vi "Config.vi"(8 "error in (no error)":errorcluster, 10 "Setting":variant, 11 "Keysight 5700C in":refnum<class "Keysight 5700C.lvclass">) -> (0 "error out":errorcluster, 3 "Keysight 5700C out":refnum<class "Keysight 5700C.lvclass">)   [LabVIEW 2025, in "Power Supply.lvlib" / "Keysight 5700C.lvclass"]
uses:
  Keysight 5700C.lvclass
  Keysight 5700C.lvclass/Keysight 5700C.ctl
  PS Channel/Power Supply Channel.lvclass
  PS Channel configuration/Power Supply Channel configuration.lvclass
  Users/Public/Documents/Sandia National Labs/TSS Plugin/Abstract Engine.lvlibp/Plugin/Abstract/Abstract Instrument/Channel.ctl
  Users/Public/Documents/Sandia National Labs/TSS Plugin/Abstract Engine.lvlibp/Plugin/Abstract/Abstract Instrument/Abstract Instrument.lvclass
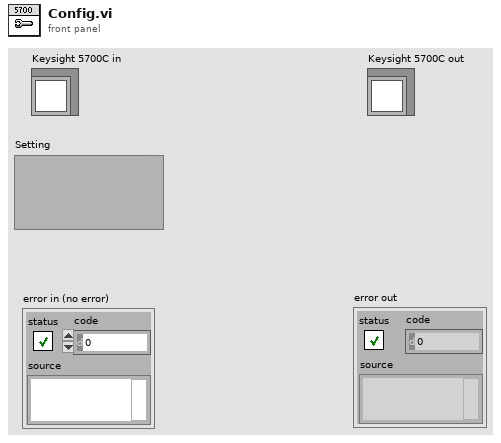
[diagram p1: front panel]
types:
  T1 = typedef "Abstract Engine.lvlibp/Abstract Instrument.lvclass/Channel.ctl" = cluster{"Alias":string, "DataType":enum16{"Anaolg Input", "Waveform"}, "Unit":enum16{"---", "V", "A", "Ohm", "Hz", "uF", "degC", "deg"}, "Upper limit":dbl, "Lower limit":dbl, "Measurement":variant}
  T2 = typedef "Abstract Engine.lvlibp/Channel configuration.lvclass/Default Channel.ctl" = cluster{"Address":string, "SW Alias":string, "Enabled":bool, "Type":string, "Description":string}
  T3 = typedef "Power Supply.lvlib/Power Supply Channel configuration.lvclass/PS Channel Setting.ctl" = cluster{"Driver":string, "Pin":string, "Test Voltage":string, "Voltage Low":dbl, "Voltage Norminal":dbl, "Voltage High":dbl, "PreTest Voltage":dbl, "PreTest Current":dbl, "Current Limit":dbl}
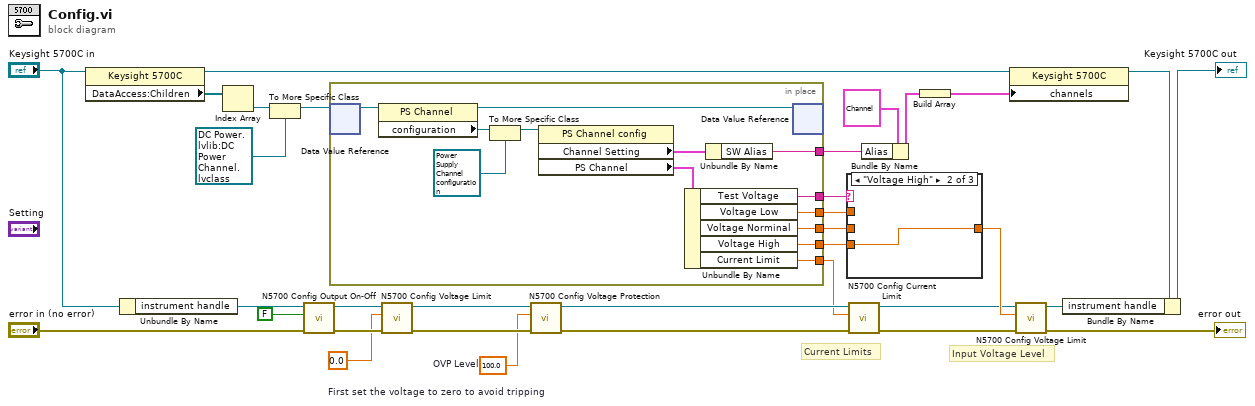
[diagram p0: block diagram]
diagram:
  w16 = 100.0  # OVP Level
  w20 = 0.0  # First set the voltage to zero to avoid tripping
  # "Input Voltage Level"
  # "Current Limits"
  n1 = property class="Keysight 5700C"(reference="Keysight 5700C in") -> (reference out=w29:refnum<class "Keysight 5700C.lvclass">, "DataAccess:Children"=w18:refnum<data-value>[])  [unwired: 1 in, 1 out]
  n2 = Unbundle By Name("Keysight 5700C in") -> ("instrument handle"=w32:refnum<visa-resource-name>)
  n3 = Index Array(array=w18) -> (element=w17:refnum<data-value>)  [unwired: 1 in]
  n4 = To More Specific Class(target class=refnum<data-value> refnum ("data value reference"), reference=w17) -> (specific class reference=w27:refnum<data-value>)  [unwired: 1 in, 1 out]
  n5 = call <instrlib>:"N5700 Config Output On-Off.vi"("error"="error in (no error)", "Output ON"=FALSE ("enabled (True)"), "VISA"=w32) -> ("error out"=w21:errorcluster, "VISA out"=w25:refnum<visa-resource-name>)  [unwired: 4 in]
  n6 = in-place {
    in-place-border: [w39] -> w13
    in-place-border: [w38] -> w12
    in-place-border: [w37] -> w11
    in-place-border: [w36] -> w10
    in-place-border: [w35] -> w9
    in-place-border: [w34] -> w8
    # "Initialize the front panel controls when loaded"
    n7 = in-place-dvr #1(w27) -> (w46:refnum<class "Power Supply Channel.lvclass">)  [unwired: 1 out]
    n8 = property class="PS Channel"(reference=w46) -> (reference out=w45:refnum<class "Power Supply Channel.lvclass">, "configuration"=w44:refnum<class "CEF_serializable configuration.lvclass">)  [unwired: 1 in, 1 out]
    n9 = To More Specific Class(target class=refnum<class "Power Supply Channel configuration.lvclass"> refnum ("DC Power.lvlib:DCPower Channel configuration.lvclass"), reference=w44) -> (specific class reference=w43:refnum<class "Power Supply Channel configuration.lvclass">)  [unwired: 1 in, 1 out]
    n10 = property class="PS Channel config"(reference=w43) -> ("Channel Setting"=w41:T2, "PS Channel"=w40:T3)  [unwired: 1 in, 2 out]
    n11 = Unbundle By Name(w40) -> ("Test Voltage"=w38:string, "Voltage Low"=w37:dbl, "Voltage Norminal"=w36:dbl, "Voltage High"=w35:dbl, "Current Limit"=w34:dbl)
    n12 = Unbundle By Name(w41) -> ("SW Alias"=w39:string)
    n13 = in-place-dvr #1(w45) -> ()  [unwired: 2 out]
  }
  n14 = call <instrlib>:"N5700 Config Voltage Limit.vi"("error"=w21, "Volt Limit"=w20, "VISA"=w25) -> ("error out"=w23:errorcluster, "VISA out"=w24:refnum<visa-resource-name>)  [unwired: 4 in]
  n15 = call <instrlib>:"N5700 Config Voltage Protection.vi"("error"=w23, "OVP Level"=w16, "VISA"=w24) -> ("error out"=w22:errorcluster, "VISA out"=w26:refnum<visa-resource-name>)  [unwired: 4 in]
  n16 = case shown="\"Voltage High\"" w12 {
    tunnel: w11 -> [_ _ w49]
    tunnel: w10 -> [w47 _ _]
    tunnel: w9 -> [_ w48 _]
    tunnel: [w47 w48 w49] -> w5
    frame "Voltage Norminal", Default {
    }
    frame "Voltage High" {
    }
    frame "Voltage Low" {
    }
  }
  n17 = call <instrlib>:"N5700 Config Current Limit.vi"("error"=w22, "Current Limit"=w8, "VISA"=w26) -> ("error out"=w7:errorcluster, "VISA out"=w4:refnum<visa-resource-name>)  [unwired: 4 in]
  n18 = Bundle By Name(cluster=T1 {"Alias"="ch0", "DataType"=enum."Anaolg Input", "Unit"=enum."V", "Upper limit"=10.0, "Lower limit"=-10.0, "Measurement"=variant} ("Channel"), "Alias"=w13) -> (w14:T1)
  n19 = Build Array(w14) -> (w2:T1[])
  n20 = property class="Keysight 5700C"(reference=w29, "channels"=w2) -> (reference out=w15:refnum<class "Keysight 5700C.lvclass">)  [unwired: 1 in, 1 out]
  n21 = call <instrlib>:"N5700 Config Voltage Limit.vi"("error"=w7, "Volt Limit"=w5, "VISA"=w4) -> ("error out"=→"error out":errorcluster, "VISA out"=w3:refnum<visa-resource-name>)  [unwired: 4 in]
  n22 = Bundle By Name(cluster=w15, "instrument handle"=w3) -> (→"Keysight 5700C out":refnum<class "Keysight 5700C.lvclass">)
